vi "SetLineVector.vi"(0 "object in":refnum<class "Align.lvclass">, 1 "lineVector":dbl[](array[numeric]), 5 "error in (no error)":errorcluster) -> (14 "object out":refnum<class "Align.lvclass">, 19 "error out":errorcluster)   [LabVIEW 2022 SP3, in "Align.lvclass"]
uses:
  Align.lvclass
  Align.lvclass/Align.ctl
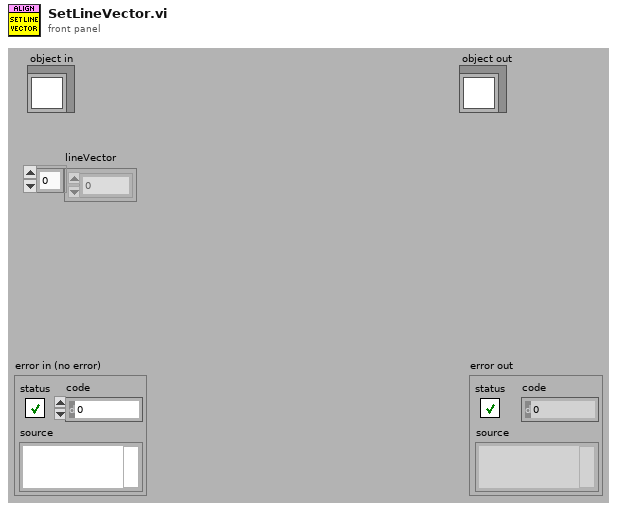
[diagram p1: front panel]
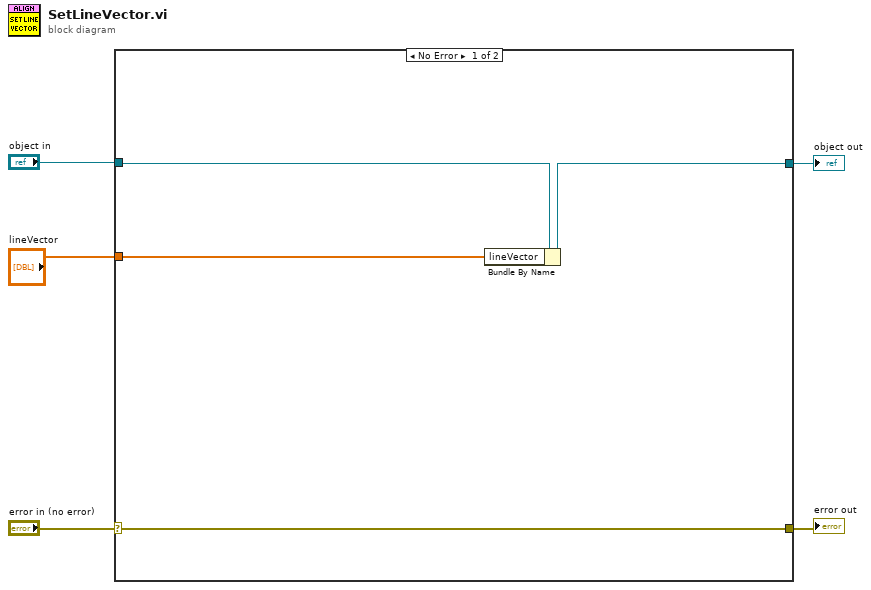
[diagram p0: block diagram]
diagram:
  n1 = case shown="No Error" "error in (no error)" {
    selector: "error in (no error)" -> [w8 w11]
    tunnel: [w8 w11] -> w4
    tunnel: [w6 w10] -> w2
    tunnel: "object in" -> [w7 w10]
    tunnel: "lineVector" -> [w9 _]
    frame No Error {
      n2 = Bundle By Name(cluster=w7, "lineVector"=w9) -> (w6:refnum<class "Align.lvclass">)
    }
    frame Error {
    }
  }
  "error out" <- w4
  "object out" <- w2
